vi "open camera settings.vi"(8 "error in (no error)":errorcluster, 11 "IMAQdx Actor in":refnum<class "IMAQdx Actor.lvclass">) -> (0 "error out":errorcluster, 3 "IMAQdx Actor out":refnum<class "IMAQdx Actor.lvclass">)   [LabVIEW 2014, in "IMAQdx Actor.lvlib" / "IMAQdx Actor.lvclass"]
uses:
  IMAQdx Actor.lvclass
  Camera Settings Dialog/Camera Settings Dialog/Camera Settings Dialog.lvclass
  IMAQdx Actor.lvclass/IMAQdx Actor.ctl
  Camera Settings Dialog/Camera Settings Dialog/Camera Settings Dialog.lvclass/Camera Settings Dialog.ctl
  <vilib>/ActorFramework/Message Enqueuer/Message Enqueuer.lvclass/Message Enqueuer.ctl
  Camera Settings Dialog/Camera Settings Dialog/Write IMAQdx Session.vi
  <vilib>/ActorFramework/Message Enqueuer/Enqueue.vi
  <vilib>/ActorFramework/Message Priority Queue/Priority Enqueue.vi
  Shared Code/Viewable Actor/ViewableActor Messages/Open Front Panel Msg/Open Front Panel Msg.lvclass
  <vilib>/ActorFramework/Actor/Actor.lvclass
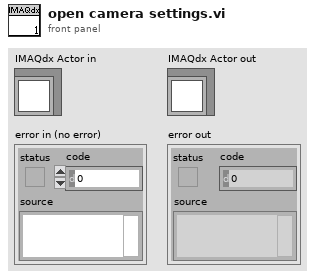
[diagram p1: front panel]
types:
  T1 = typedef "IMAQdx.ctl" = refnum<k21>
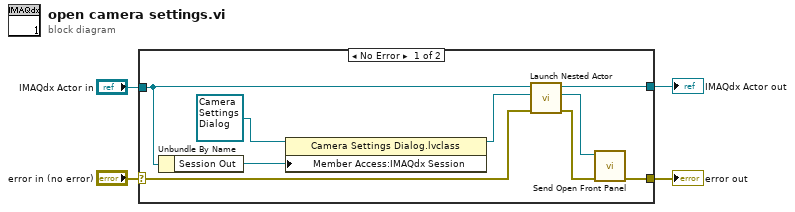
[diagram p0: block diagram]
diagram:
  n1 = case shown="No Error" "error in (no error)" {
    selector: "error in (no error)" -> [w8 w15]
    tunnel: [w5 w15] -> w3
    tunnel: [w13 w14] -> w1
    tunnel: "IMAQdx Actor in" -> [w10 w14]
    frame No Error {
      n2 = Unbundle By Name(w10) -> ("Session Out"=w9:T1)
      n3 = property class="Camera Settings Dialog.lvclass"(reference=refnum<class "Camera Settings Dialog.lvclass"> refnum ("Camera Settings Dialog.lvlib:Camera Settings Dialog.lvclass"), "Member Access:IMAQdx Session"=w9) -> (reference out=w11:refnum<class "Camera Settings Dialog.lvclass">)  [unwired: 1 in, 1 out]
      n4 = call <vilib>:"Launch Nested Actor.vi"("error in (no error)"=w8, "Nested Actor"=w11, "Caller Actor in"=w10) -> ("error out"=w6:errorcluster, "Nested Actor's Enqueuer"=w7:refnum<class "Message Enqueuer.lvclass">, "Caller Actor out"=w13:refnum<class "IMAQdx Actor.lvclass">)  [unwired: 6 in]
      n5 = call "Send Open Front Panel.vi"("error in (no error)"=w6, "Message Enqueuer"=w7) -> ("error out"=w5:errorcluster)  [unwired: 8 in, 1 out]
    }
    frame Error {
    }
  }
  "error out" <- w3
  "IMAQdx Actor out" <- w1
